vi "ParametersToState.vi"(0 "ParametersToState":T4, 7 "StateIn":T1 {"ILoad" format="%_6g"; "Fault Registers" format="%016x"; "VLoad" format="%_6g"; "VDCLink" format="%_6g"; "Detected Frequency" format="%1_6g"}) -> (8 "StateOut":T1 {"ILoad" format="%_6g"; "Fault Registers" format="%016x"; "VLoad" format="%_6g"; "VDCLink" format="%_6g"; "Detected Frequency" format="%1_6g"})   [LabVIEW 2017, in "AppStateMachine runtime.lvclass"]
uses:
  AppStateMachine runtime.lvclass
  parameter user data.ctl
  State.ctl
  StateId.ctl
  LED_Color.ctl
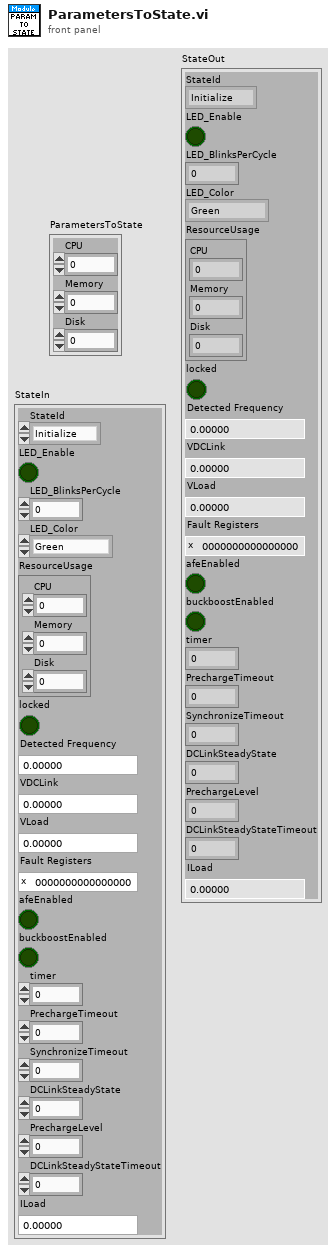
[diagram p1: front panel]
types:
  T1 = typedef "AppStateMachine runtime.lvclass/State.ctl" = cluster{"StateId":T2, "LED_Enable":bool, "LED_BlinksPerCycle":i32, "LED_Color":T3, "ResourceUsage":cluster{"CPU":dbl, "Memory":dbl, "Disk":dbl}, "locked":bool, "Detected Frequency":dbl, "VDCLink":dbl, "VLoad":dbl, "Fault Registers":u64, "afeEnabled":bool, "buckboostEnabled":bool, "timer":u32, "PrechargeTimeout":u32, "SynchronizeTimeout":u32, "DCLinkSteadyState":dbl, "PrechargeLevel":dbl, "DCLinkSteadyStateTimeout":u32, "ILoad":dbl}
  T2 = typedef "AppStateMachine runtime.lvclass/StateId.ctl" = enum16{"Initialize", "Idle", "TunePLL", "TuneAFE", "TuneBuckBoost", "Precharge", "Synchronize", "Ready", "EnableAFE", "EnableBuckBoost", "Powered", "SafeState", "UnrecoverableSafeState"}
  T3 = typedef "AppStateMachine runtime.lvclass/LED_Color.ctl" = enum16{"Green", "Yellow"}
  T4 = typedef "AppStateMachine runtime.lvclass/parameter user data.ctl" = cluster{"CPU":dbl, "Memory":dbl, "Disk":dbl}
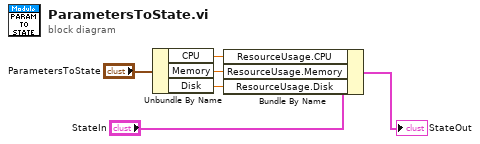
[diagram p0: block diagram]
diagram:
  n1 = Unbundle By Name("ParametersToState") -> ("CPU"=w3:dbl, "Memory"=w2:dbl, "Disk"=w1:dbl)
  n2 = Bundle By Name(cluster="StateIn", "ResourceUsage.CPU"=w3, "ResourceUsage.Memory"=w2, "ResourceUsage.Disk"=w1) -> (→"StateOut":T1)
